vi "HRV_Analysis.vi"(1 "Frame Length":i32=100, 2 "Sample Rate":dbl=500.0 format="%#_13g", 3 "PPG_Data":dbl[](array[numeric])) -> (0 "ln (VLF, HF)":dbl[](array[numeric]))   [LabVIEW 2014]
uses:
  <vilib>/Analysis/1siggen.llb/Ramp Pattern by Samples.vi
  <vilib>/Analysis/NI_AAL_SigProc.lvlib
  <vilib>/Analysis/NI_AALBase.lvlib
  <vilib>/Analysis/NI_AALPro.lvlib
  <vilib>/gmath/NI_Gmath.lvlib
panel:
  out "XY 그래프":cluster{"Ramp Pattern":dbl[], dbl[]}[](graph)=[{"Ramp Pattern"=array[1200 elements], array[1200 elements]}, {"Ramp Pattern"=[208.0, 467.0, 739.0, 964.5], [0.15519410837197323, 0.2060507413617612, 0.20663103640135128, 0.1694172665872692]}, {"Ramp Pattern"=[191.0, 225.0, 453.0, 483.0, 727.0, 758.0, 923.0, 1009.0], [0.0, 0.05511811023622047, 0.11023622047244094, 0.16535433070866143, 0.2204724409448819, 0.2755905511811024, 0.33070866141732286, 0.3858267716535433, 0.4409448818897638, 0.49606299212598426, 0.5511811023622047, 0.6062992125984252, 0.6614173228346457, 0.7165354330708661, 0.7716535433070866, 0.8267716535433071, 0.8818897637795275, 0.937007874015748, 0.9921259842519685, 1.047244094488189, 1.1023622047244095, 1.1574803149606299, 1.2125984251968505, 1.2677165354330708, 1.3228346456692914, 1.3779527559055118, 1.4330708661417322, 1.4881889763779528, 1.5433070866141732, 1.5984251968503937, 1.6535433070866141, 1.7086614173228347, 1.763779527559055, 1.8188976377952757, 1.874015748031496, 1.9291338582677164, 1.984251968503937, 2.0393700787401574, 2.094488188976378, 2.1496062992125986, 2.204724409448819, 2.2598425196850394, 2.3149606299212597, 2.37007874015748, 2.425196850393701, 2.4803149606299213, 2.5354330708661417, 2.590551181102362, 2.645669291338583, 2.7007874015748032, 2.7559055118110236, 2.811023622047244, 2.8661417322834644, 2.921259842519685, 2.9763779527559056, 3.031496062992126, 3.0866141732283463, 3.141732283464567, 3.1968503937007875, 3.251968503937008, 3.3070866141732282, 3.3622047244094486, 3.4173228346456694, 3.47244094488189, 3.52755905511811, 3.5826771653543306, 3.6377952755905514, 3.6929133858267718, 3.748031496062992, 3.8031496062992125, 3.858267716535433, 3.9133858267716537, 3.968503937007874, 4.0236220472440944, 4.078740157480315, 4.133858267716535, 4.188976377952756, 4.244094488188976, 4.299212598425197, 4.354330708661418, 4.409448818897638, 4.464566929133858, 4.519685039370079, 4.574803149606299, 4.6299212598425195, 4.68503937007874, 4.74015748031496, 4.7952755905511815, 4.850393700787402, 4.905511811023622, 4.960629921259843, 5.015748031496063, 5.070866141732283, 5.125984251968504, 5.181102362204724, 5.2362204724409445, 5.291338582677166, 5.346456692913386, 5.4015748031496065, 5.456692913385827, 5.511811023622047, 5.566929133858268, 5.622047244094488, 5.677165354330708, 5.732283464566929, 5.78740157480315, 5.84251968503937, 5.897637795275591, 5.952755905511811, 6.0078740157480315, 6.062992125984252, 6.118110236220472, 6.173228346456693, 6.228346456692913, 6.283464566929134, 6.338582677165355, 6.393700787401575, 6.448818897637795, 6.503937007874016, 6.559055118110236, 6.6141732283464565, 6.669291338582677, 6.724409448818897, 6.7795275590551185, 6.834645669291339, 6.889763779527559, 6.94488188976378, 7.0]}]
  out "mean":dbl format="%0.2f"
  out "SDNN":dbl
  out "PPI":dbl
  out "BPM":dbl
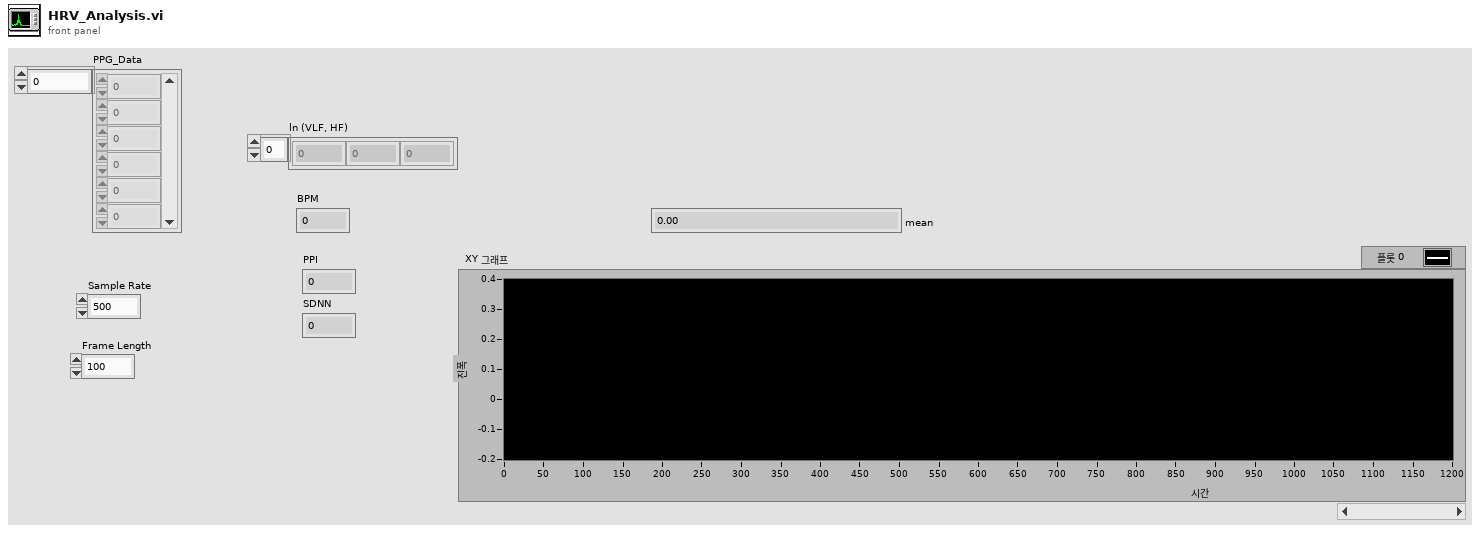
[diagram p1: front panel]
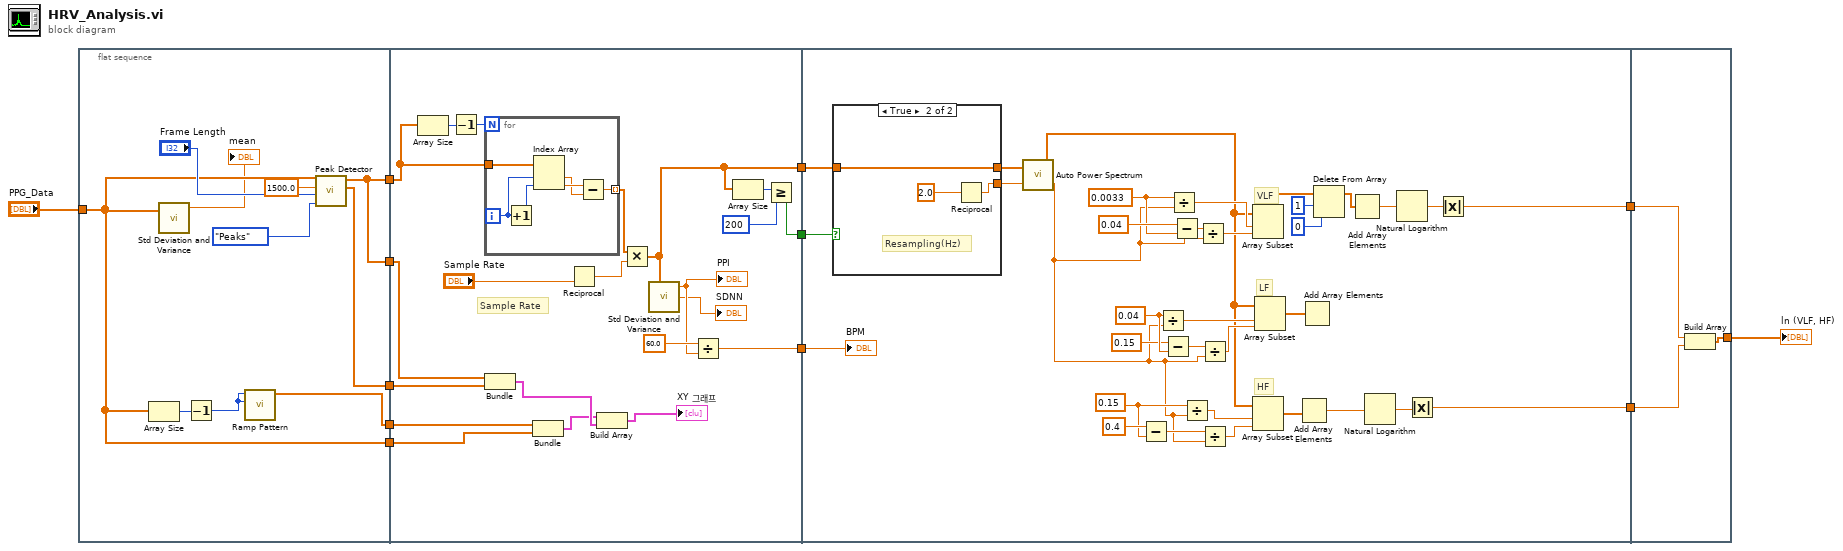
[diagram p0: block diagram]
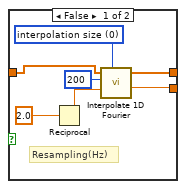
[diagram p2: hidden frame]
diagram:
  n1 = flat-sequence {
    tunnel: [w19] -> w12
    tunnel: "PPG_Data" -> [w17]
    tunnel: [w17] -> w4
    tunnel: [w20] -> w3
    tunnel: [w19] -> w2
    tunnel: [w16] -> w1
    tunnel: w12 -> [w41]
    tunnel: [w36] -> w11
    tunnel: [w33] -> w10
    tunnel: [w31] -> w7
    tunnel: w4 -> [w26]
    tunnel: w3 -> [w29]
    tunnel: w2 -> [w28]
    tunnel: w1 -> [w25]
    tunnel: w11 -> [w60]
    tunnel: w10 -> [w57]
    tunnel: w7 -> [w56]
    tunnel: [w51] -> w6
    tunnel: [w50] -> w5
    tunnel: [w96] -> w9
    tunnel: w6 -> [w95]
    tunnel: w5 -> [w94]
    frame #0 {
      n2 = Array Size(array=w17) -> (size(s)=w18:i32)
      n3 = call <vilib>:"Std Deviation and Variance.vi"("X"=w17) -> ("mean"=→"mean":dbl)  [unwired: 1 in, 2 out]
      n4 = Decrement(x=w18) -> (x-1=w15:i32)
      n5 = call-poly <vilib>:"Ramp Pattern.vi"("end"=w15, "samples"=w15) -> ("Ramp Pattern"=w16:dbl[])  [unwired: 8 in, 1 out]
      n6 = call <vilib>:"Peak Detector.vi"("peaks/valleys"=enum32{"Peaks", "Valleys"}."Peaks", "width"="Frame Length", "threshold"=1500.0, "X"=w17) -> ("Amplitudes"=w20:dbl[], "Locations"=w19:dbl[])  [unwired: 3 in, 3 out]
    }
    frame #1 {
      # "Sample Rate"
      n7 = Array Size(array=w41) -> (size(s)=w43:i32)
      n8 = Decrement(x=w43) -> (x-1=w42:i32)
      n9 = for {
        N: w42 -> [_]
        tunnel: w41 -> [w49]
        tunnel: [w44] -> w40 mode=indexing
        i -> [w47]
        n10 = Increment(x=w47) -> (x+1=w48:i32)
        n11 = Index Array(array=w49, index #1=w47, index #2=w48) -> (element #1=w45:dbl, element #2=w46:dbl)
        n12 = Subtract(x=w46, y=w45) -> (x-y=w44:dbl)
      }
      n13 = Bundle("Locations"=w28, "Amplitudes"=w29) -> (w27:cluster{"Locations":dbl[], "Amplitudes":dbl[]})  [unwired: 1 in]
      n14 = Bundle("Ramp Pattern"=w25, "PPG_Data"=w26) -> (w24:cluster{"Ramp Pattern":dbl[], "PPG_Data":dbl[]})  [unwired: 1 in]
      n15 = Reciprocal(x="Sample Rate") -> (1/x=w39:dbl)
      n16 = Build Array(w24, w27) -> (→"XY 그래프":cluster{"Locations":dbl[], "Amplitudes":dbl[]}[])
      n17 = Multiply(x=w40, y=w39) -> (x*y=w36:dbl[])
      n18 = call <vilib>:"Std Deviation and Variance.vi"("X"=w36) -> ("mean"=w32:dbl, "standard deviation"=→"SDNN":dbl)  [unwired: 1 in, 1 out]
      "PPI" <- w32
      n19 = Divide(x=60.0, y=w32) -> (x/y=w31:dbl)
      n20 = Array Size(array=w36) -> (size(s)=w35:i32)
      n21 = Greater Or Equal?(x=w35, y=200) -> (x >= y?=w33:bool)
    }
    frame #2 {
      w71 = 0.0033 ("x")
      w76 = 0.15 ("x")
      w82 = 0.04 ("x")
      # "VLF"
      # "HF"
      # "LF"
      n22 = case shown="True" w57 {
        tunnel: w60 -> [w86 w92]
        tunnel: [w85 w91] -> w59
        tunnel: [w84 w92] -> w58
        frame False {
          w88 = u16 0 items=["interpolation size", "interpolation factor"] ("type")
          # "Resampling(Hz)"
          n23 = Reciprocal(x=2.0 ("Resampling(Hz)")) -> (1/x=w89:dbl)
          n24 = call <vilib>:"Interpolate 1D Fourier.vi"("type"=w88, "dt in"=w89, "n"=200, "X"=w86) -> ("dt out"=w85:dbl, "Y"=w84:dbl[])  [unwired: 4 in, 2 out]
        }
        frame True {
          # "Resampling(Hz)"
          n25 = Reciprocal(x=2.0 ("Resampling(Hz)")) -> (1/x=w91:dbl)
        }
      }
      n26 = call <vilib>:"Auto Power Spectrum.vi"("dt"=w59, "Signal (V)"=w58) -> ("df"=w61:dbl, "Power Spectrum (V^2 rms)"=w62:dbl[])
      n27 = Subtract(x=0.4, y=w76) -> (x-y=w78:dbl)
      n28 = Divide(x=w82, y=w61) -> (x/y=w83:dbl)
      n29 = Subtract(x=0.15, y=w82) -> (x-y=w80:dbl)
      n30 = Divide(x=w71, y=w61) -> (x/y=w70:dbl)
      n31 = Subtract(x=0.04, y=w71) -> (x-y=w73:dbl)
      n32 = Divide(x=w76, y=w61) -> (x/y=w75:dbl)
      n33 = Divide(x=w73, y=w61) -> (x/y=w69:dbl)
      n34 = Divide(x=w80, y=w61) -> (x/y=w79:dbl)
      n35 = Divide(x=w78, y=w61) -> (x/y=w74:dbl)
      n36 = Array Subset(array=w62, index=w70, length=w69) -> (w64:dbl[])
      n37 = Array Subset(array=w62, index=w75, length=w74) -> (w67:dbl[])
      n38 = Array Subset(array=w62, index=w83, length=w79) -> (w68:dbl[])
      n39 = Add Array Elements(numeric array=w67) -> (sum=w52:dbl)
      n40 = Add Array Elements(numeric array=w68) -> ()  [unwired: 1 out]
      n41 = Delete From Array(array=w64, length=1 ("길이"), index=0 ("인덱스")) -> (array with subset deleted=w63:dbl[])  [unwired: 1 out]
      n42 = Add Array Elements(numeric array=w63) -> (sum=w54:dbl)
      n43 = Natural Logarithm(1:w52) -> (0:w53:dbl)
      n44 = Natural Logarithm(1:w54) -> (0:w55:dbl)
      n45 = Absolute Value(x=w53) -> (abs(x)=w50:dbl)
      n46 = Absolute Value(x=w55) -> (abs(x)=w51:dbl)
      "BPM" <- w56
    }
    frame #3 {
      n47 = Build Array(w95, w94) -> (w96:dbl[])
    }
  }
  "ln (VLF, HF)" <- w9
